vi "DriveModuleControl.vi"(8 "error in":errorcluster, 9 "Actual State":T1={"Speed"=0.0, "Angle"={"VALUE"=0.0, "COS"=1.0, "SIN"=0.0}} {"Angle"."SIN" format="%13.4f"; "Angle"."COS" format="%13.4f"; "Angle"."VALUE" format="%13.4f"}, 10 "Desired State":T1={"Speed"=0.0, "Angle"={"VALUE"=0.0, "COS"=1.0, "SIN"=0.0}} {"Angle"."SIN" format="%13.4f"; "Angle"."COS" format="%13.4f"; "Angle"."VALUE" format="%13.4f"}, 11 "ModualNamePrefix":i32) -> (0 "error out":errorcluster)   [LabVIEW 2020]
uses:
  <vilib>/Rock Robotics/WPI/ThirdParty/JAS_Junk/TrajLib/TypeDef/SWERVE_DRIVE_MODULE_STATE.ctl
  <vilib>/Rock Robotics/WPI/ThirdParty/JAS_Junk/TrajLib/TypeDef/ROTATION2D.ctl
  <vilib>/Rock Robotics/WPI/ThirdParty/JAS_Junk/TrajLib/Rotation2d_Minus.vi
  <vilib>/Rock Robotics/WPI/ThirdParty/JAS_Junk/TrajLib/Rotation2d_GetRadians.vi
  <vilib>/Rock Robotics/WPI/ThirdParty/JAS_Junk/TrajLib/SwerveModuleState_New.vi
  <vilib>/Rock Robotics/WPI/ThirdParty/JAS_Junk/TrajLib/Rotation2d_RotateBy.vi
  <vilib>/Rock Robotics/WPI/ThirdParty/JAS_Junk/TrajLib/Rotation2d_CreateAngle.vi
  <vilib>/Rock Robotics/WPI/ThirdParty/JAS_Junk/TrajLib/SimpleMotorFF_Calculate.vi
  <vilib>/Rock Robotics/WPI/ThirdParty/JAS_Junk/TrajLib/PIDController_AtSetpoint.vi
  <vilib>/Rock Robotics/WPI/ThirdParty/JAS_Junk/TrajLib/PIDController_SetPIDF.vi
  <vilib>/Rock Robotics/WPI/ThirdParty/JAS_Junk/TrajLib/PIDController_SetDerivativeFilter.vi
  <vilib>/Rock Robotics/WPI/ThirdParty/JAS_Junk/TrajLib/PIDController_SetIntegratorRange.vi
  <vilib>/Rock Robotics/WPI/ThirdParty/JAS_Junk/TrajLib/PIDController_SetTolerancePandV.vi
  <vilib>/Rock Robotics/WPI/ThirdParty/JAS_Junk/TrajLib/PIDController_DisableContinousInput.vi
  <vilib>/Rock Robotics/WPI/ThirdParty/JAS_Junk/TrajLib/PIDController_EnableContinousInput.vi
  <vilib>/Rock Robotics/WPI/ThirdParty/JAS_Junk/TrajLib/PIDController_Reset.vi
  <vilib>/Rock Robotics/WPI/ThirdParty/JAS_Junk/TrajLib/PIDController_New.vi
  <vilib>/Rock Robotics/WPI/ThirdParty/JAS_Junk/TrajLib/PIDController_SetOutputLimits.vi
  <vilib>/Rock Robotics/WPI/ThirdParty/JAS_Junk/TrajLib/Rotation2d_UnaryMinus.vi
  <vilib>/Rock Robotics/WPI/ThirdParty/JAS_Junk/TrajLib/Rotation2d_CreateXY.vi
  <vilib>/Rock Robotics/WPI/ThirdParty/JAS_Junk/TrajLib/PIDController_NewPeriod.vi
  <vilib>/Rock Robotics/WPI/ThirdParty/JAS_Junk/TrajLib/Util_CalcDist.vi
  <vilib>/Rock Robotics/SystemInterfaces/NetworkCommunication/NetComm_UsageReport_report.vi
  DriveGlobal.vi
  <vilib>/Rock Robotics/WPI/ThirdParty/JAS_Junk/TrajLib/Globals/Util_LibraryGlobals.vi
  <vilib>/Rock Robotics/WPI/ThirdParty/JAS_Junk/TrajLib/PIDController_AdvCalculate_FF_Sp_Pv.vi
  <vilib>/Rock Robotics/Network Tables/NT Write Number.vi
  <vilib>/Rock Robotics/WPI/ThirdParty/JAS_Junk/TrajLib/Trajectory_Library.lvlib
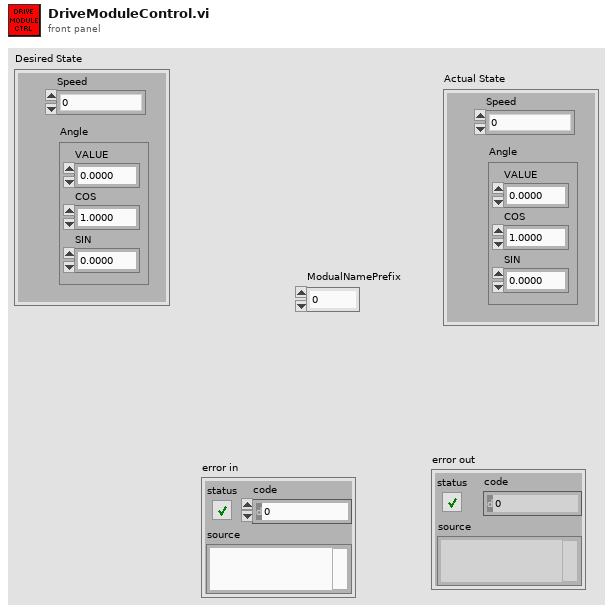
[diagram p1: front panel]
types:
  T1 = typedef "Trajectory_Library.lvlib/SWERVE_DRIVE_MODULE_STATE.ctl" = cluster{"Speed":dbl, "Angle":T2}
  T2 = typedef "Trajectory_Library.lvlib/ROTATION2D.ctl" = cluster{"VALUE":dbl, "COS":dbl, "SIN":dbl}
  T3 = typedef "WPI_MotorControlDeviceRef.ctl" = cluster{"DeviceStatus":errorcluster, "Type":T4, "PWM":cluster{"PWM Channel":T5, "DeadBand":T6}, "CAN":cluster{"Device Number":u8, "SetOutput VI Ref":variant, "GetOutput VI Ref":variant, "Enable VI Ref":variant, "Disable VI Ref":variant, "Data":variant}, "Invert":bool, "DIO PWM":cluster{"PWM \"Enable\" Channel":T5, "DIOChannel":T7, "PWM Rate":dbl}}
  T4 = typedef "WPI_MotorControlType.ctl" = enum16{"PWM", "CAN", "DIO PWM"}
  T5 = typedef "FPGA_DIOPWMChannel.ctl" = enum8{"PWM 0", "PWM 1", "PWM 2", "PWM 3", "PWM 4", "PWM 5", "PWM 6", "PWM 7", "PWM 8", "PWM 9", "PWM MXP 0", "PWM MXP 1", "PWM MXP 2", "PWM MXP 3", "PWM MXP 4", "PWM MXP 5", "PWM MXP 6", "PWM MXP 7", "PWM MXP 8", "PWM MXP 9", "Invalid"}
  T6 = typedef "WPI_PWMDeadband.ctl" = cluster{"Name":string, "maxPositivePwm":i32, "minPositivePwm":i32, "centerPwm":i32, "maxNegativePwm":i32, "minNegativePwm":i32, "angularRange":u16}
  T7 = typedef "FPGA_DIOChannel.ctl" = enum8{"DIO 0", "DIO 1", "DIO 2", "DIO 3", "DIO 4", "DIO 5", "DIO 6", "DIO 7", "DIO 8", "DIO 9", "DIO MXP 0", "DIO MXP 1", "DIO MXP 2", "DIO MXP 3", "DIO MXP 4", "DIO MXP 5", "DIO MXP 6", "DIO MXP 7", "DIO MXP 8", "DIO MXP 9", "DIO MXP 10", "DIO MXP 11", "DIO MXP 12", "DIO MXP 13", "DIO MXP 14", "DIO MXP 15", "SPI Port CS1", "SPI Port CS2", "SPI Port CS3", "SPI Port MISO", "SPI Port MOSI", "Invalid"}
  T8 = typedef "Trajectory_Library.lvlib/SIMPLE_MOTOR_FF.ctl" = cluster{"Ks":dbl, "Kv":dbl, "Ka":dbl, "KnInv":dbl}
  T9 = typedef "Trajectory_Library.lvlib/PID_ADV_LIMITS.ctl" = cluster{"MaxInput":dbl, "MinInput":dbl, "Continuous":bool, "MaxOutput":dbl, "MinOutput":dbl}
  T10 = typedef "Trajectory_Library.lvlib/PID_ADV_TUNING.ctl" = cluster{"Kf":dbl, "Kp":dbl, "Ki":dbl, "Kd":dbl, "MaximumIntegral":dbl, "MinimumIntegral":dbl, "Filter Derivative":bool}
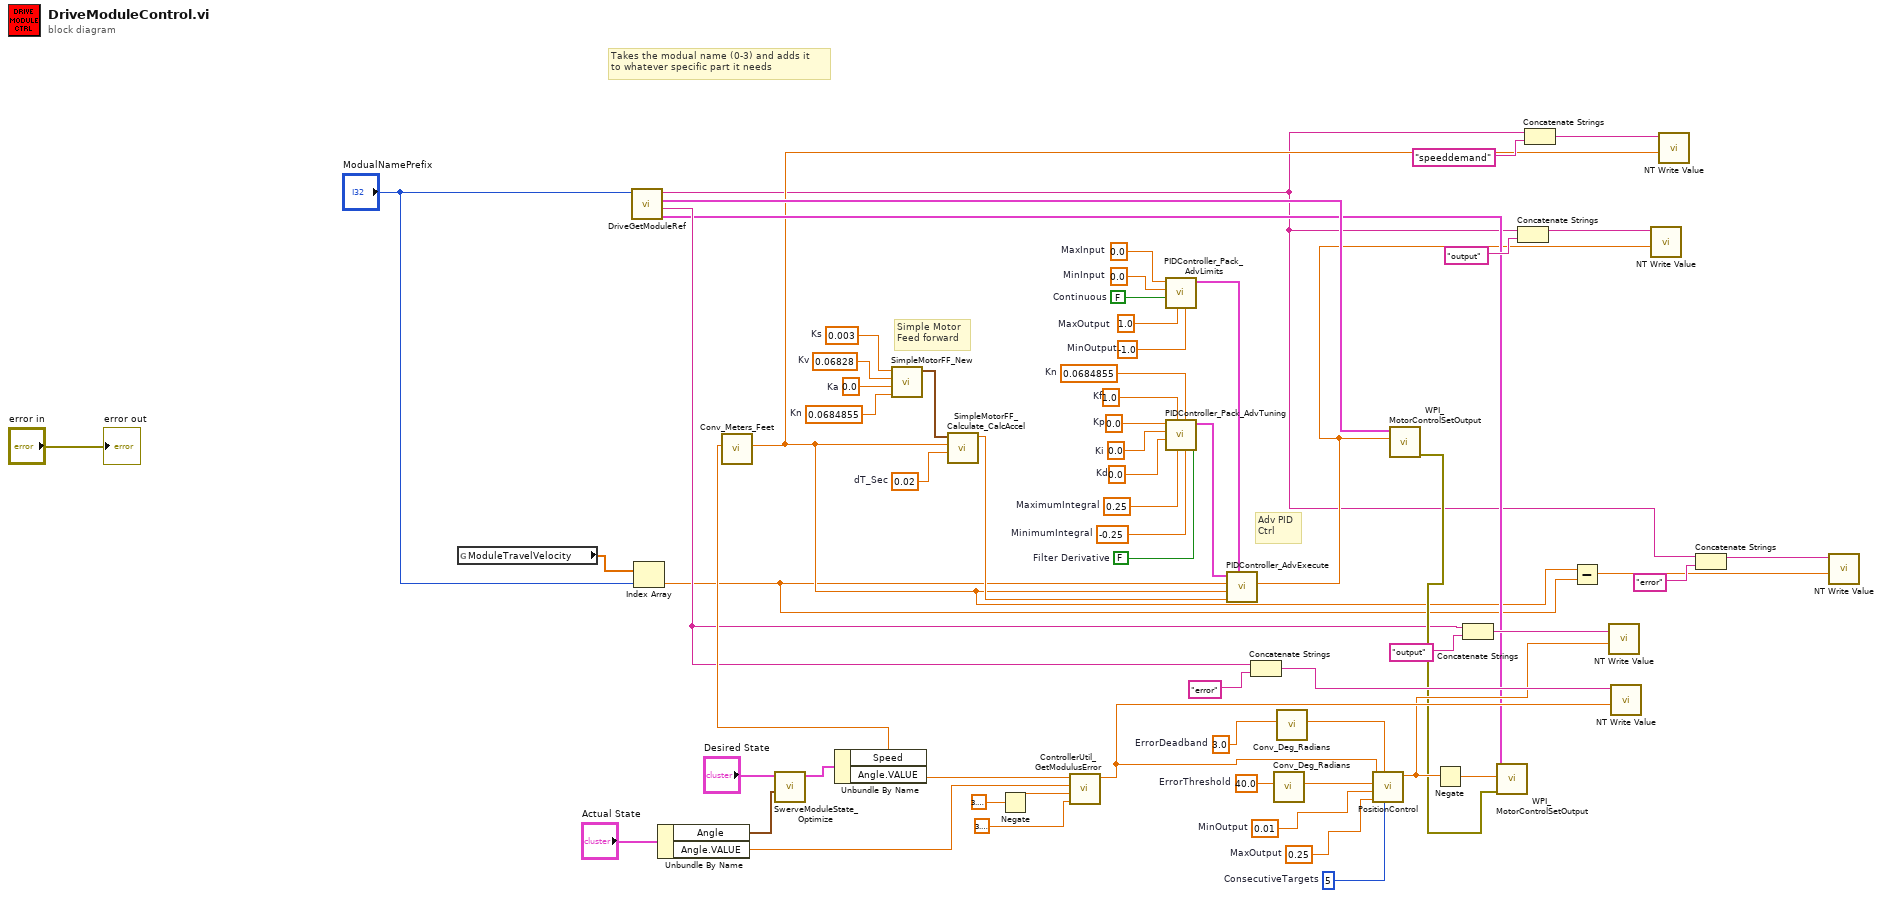
[diagram p0: block diagram]
diagram:
  w7 = 0.0684855  # Kn
  w25 = 0.0  # Kp
  w24 = 0.0  # Ki
  w23 = 0.0  # Kd
  w22 = 1.0  # Kf
  w21 = 0.25  # MaximumIntegral
  w20 = -0.25  # MinimumIntegral
  w19 = FALSE  # Filter Derivative
  w17 = 0.0  # MinInput
  w16 = FALSE  # Continuous
  w15 = 1.0  # MaxOutput
  w18 = -1.0  # MinOutput
  w14 = 0.0  # MaxInput
  w35 = 0.0684855  # Kn
  w34 = 0.02  # dT_Sec
  w32 = 0.003  # Ks
  w31 = 0.06828  # Kv
  w30 = 0.0  # Ka
  w46 = 5  # ConsecutiveTargets
  w43 = 0.25  # MaxOutput
  w47 = 0.01  # MinOutput
  w40 = 40.0  # ErrorThreshold
  w42 = 3.0  # ErrorDeadband
  # "Adv PID\nCtrl"
  # "Simple Motor\nFeed forward"
  # "Takes the modual name (0-3) and adds it \nto whatever specific part it needs"
  n1 = global read "DriveGlobal.vi" "ModuleTravelVelocity"() -> (w9:dbl[])
  n2 = call "DriveGetModuleRef.vi"("ModualNamePrefix"="ModualNamePrefix") -> ("SpinMot"=w26:T3, "SpinStr"=w27:string, "TravMot"=w28:T3, "TravStr"=w1:string)  [unwired: 5 in, 2 out]
  n3 = Index Array(array=w9, index="ModualNamePrefix") -> (element=w5:dbl)
  n4 = Unbundle By Name("Actual State") -> ("Angle"=w54:T2, "Angle.VALUE"=w50:dbl)
  n5 = call <vilib>:"SwerveModuleState_Optimize.vi"("CurrentAngle"=w54, "Desired State"="Desired State") -> ("out SWERVE_DRIVE_MODULE_STATE"=w52:T1)  [unwired: 9 in]
  n6 = Unbundle By Name(w52) -> ("Speed"=w36:dbl, "Angle.VALUE"=w51:dbl)
  n7 = call <vilib>:"Conv_Meters_Feet.vi"("Meters"=w36) -> ("Feet"=w6:dbl)  [unwired: 10 in]
  n8 = call <vilib>:"SimpleMotorFF_New.vi"("Kn"=w35, "Ka"=w30, "Kv"=w31, "Ks"=w32) -> ("SIMPLE_MOTOR_FF"=w33:T8)  [unwired: 7 in]
  n9 = call <vilib>:"SimpleMotorFF_Calculate_CalcAccel.vi"("dT_Sec"=w34, "VelSp"=w6, "SIMPLE_MOTOR_FF"=w33) -> ("FeedForward"=w10:dbl)  [unwired: 8 in]
  n10 = Negate(x=3.141592653589793) -> (-x=w53:dbl)
  n11 = call <vilib>:"ControllerUtil_GetModulusError.vi"("Maximum_Input"=3.141592653589793, "Minimum_Input"=w53, "Measurerment(PV)"=w50, "Reference(SP)"=w51) -> ("Error"=w44:dbl)  [unwired: 7 in]
  n12 = call <vilib>:"PIDController_Pack_AdvLimits.vi"("MinOutput"=w18, "MaxOutput"=w15, "Continuous"=w16, "MinInput"=w17, "MaxInput"=w14) -> ("Adv PID Limits"=w12:T9)  [unwired: 6 in]
  n13 = call <vilib>:"PIDController_Pack_AdvTuning.vi"("Filter Derivative"=w19, "MinimumIntegral"=w20, "Kn"=w7, "MaximumIntegral"=w21, "Kf"=w22, "Kd"=w23, "Ki"=w24, "Kp"=w25) -> ("Adv PID Tuning"=w13:T10)  [unwired: 3 in]
  n14 = call <vilib>:"PIDController_AdvExecute.vi"("Adv PID Limits"=w12, "FF-FeedForward"=w10, "SP-SetPoint"=w6, "PV-Measurement"=w5, "Adv PID Tuning"=w13) -> ("CO-ControlOutput"=w11:dbl)  [unwired: 4 in, 2 out]
  n15 = Concatenate Strings(w27, "error" ("refnum name")) -> (w58:string)
  n16 = call <vilib>:"Conv_Deg_Radians.vi"("Degress"=w40) -> ("Radians"=w39:dbl)  [unwired: 10 in]
  n17 = call <vilib>:"Conv_Deg_Radians.vi"("Degress"=w42) -> ("Radians"=w41:dbl)  [unwired: 10 in]
  n18 = call "PositionControl.vi"("ConsecutiveTargets"=w46, "ErrorDeadband"=w41, "MaxOutput"=w43, "MinOutput"=w47, "ErrorThreshold"=w39, "Error"=w44) -> ("OutputValue"=w38:dbl)  [unwired: 3 in, 2 out]
  n19 = call <vilib>:"WPI_MotorControlSetOutput.vi"("Output"=w11, "MotorControlDevRef"=w28) -> ("error out"=w29:errorcluster)  [unwired: 7 in, 2 out]
  n20 = Negate(x=w38) -> (-x=w37:dbl)
  n21 = Concatenate Strings(w27, "output" ("refnum name")) -> (w45:string)
  n22 = call <vilib>:"WPI_MotorControlSetOutput.vi"("error in (no error)"=w29, "Output"=w37, "MotorControlDevRef"=w26) -> ()  [unwired: 6 in, 3 out]
  n23 = Concatenate Strings(w1, "output" ("refnum name")) -> (w60:string)
  n24 = Concatenate Strings(w1, "speeddemand" ("refnum name")) -> (w62:string)
  n25 = Subtract(x=w6, y=w5) -> (x-y=w2:dbl)
  n26 = call-poly <vilib>:"NT Write Value.vi"("value"=w38, "name"=w45) -> ()  [unwired: 9 in, 1 out]
  n27 = call-poly <vilib>:"NT Write Value.vi"("value"=w44, "name"=w58) -> ()  [unwired: 9 in, 1 out]
  n28 = call-poly <vilib>:"NT Write Value.vi"("value"=w11, "name"=w60) -> ()  [unwired: 9 in, 1 out]
  n29 = call-poly <vilib>:"NT Write Value.vi"("value"=w6, "name"=w62) -> ()  [unwired: 9 in, 1 out]
  n30 = Concatenate Strings(w1, "error" ("refnum name")) -> (w3:string)
  n31 = call-poly <vilib>:"NT Write Value.vi"("value"=w2, "name"=w3) -> ()  [unwired: 9 in, 1 out]
  "error out" <- "error in"
